vi "Structure Key to Name.vi"(5 "Key":string) -> (2 "Name":string)   [LabVIEW 2019]
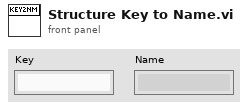
[diagram p1: front panel]
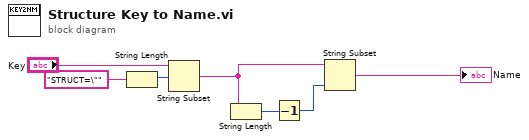
[diagram p0: block diagram]
diagram:
  n1 = String Length(string="STRUCT=\"") -> (length=w5:i32)
  n2 = String Subset(string="Key", offset (0)=w5) -> (substring=w2:string)  [unwired: 1 in]
  n3 = String Length(string=w2) -> (length=w4:i32)
  n4 = Decrement(x=w4) -> (x-1=w3:i32)
  n5 = String Subset(string=w2, length (rest)=w3) -> (substring=→"Name":string)  [unwired: 1 in]
